vi "Exercise2.3-WBFM Modulation Demo (Music) .vi"() -> ()   [LabVIEW 2013]
uses:
  <vilib>/sound2/lvsound2.llb/Sound File Info (path).vi
  <vilib>/sound2/lvsound2.llb/Sound File Read Open.vi
  <vilib>/sound2/lvsound2.llb/Sound File Read (DBL).vi
  <vilib>/Waveform/WDTOps.llb/WDT Get Waveform Subset DBL.vi
  <vilib>/addons/Modulation/Analog/MT Passband PLL.vi
  <vilib>/express/express analysis/Spectral/Block/exnSpectralBlock spectral measurements power poly.vi
  <vilib>/express/express analysis/Spectral/Block/exnSpectralBlock spectral measurements power DDT.vi
  <vilib>/express/express analysis/Spectral/XNode/ExpressSpectralMeasurementsBlockNode.xnode
  <vilib>/addons/Modulation/niAMT.lvlib
  <vilib>/Analysis/NI_AALPro.lvlib
panel:
  out "Baseband":dynamicdata(graph)
  in  "Resample Rate":dbl=1000000.0 format="%#_13g"
  in  "Duration":dbl=44101.0 format="%#_13g"
  in  "path":path=path "D:/File/mozart.wav"
  out "Estimated freq.":dbl
  in  "WAV SR":dbl=44100.0 caption="dt"
  in  "LPF Cut-Off":dbl=60000.0 caption="Lower Cut-Off"
  in  "SNR (dB)":dbl(slide)=30.0 caption="Standard deviation" scale=-20.0..100.0
  out "Recovered Signal":dynamicdata(graph)
  out "FM Spectrum":dynamicdata(graph)
  out "FM Wave":dynamicdata(graph)
  in  "Carrier Amp.":dbl=1.0 caption="Amplitude"
  in  "stop":bool
  in  "Frequency Deviation":dbl(slide)=200.0 scale=0.0..100000.0
  in  "Carrier Freq.":dbl=100000.0 caption="Frequency"
  # "Frequency Modulation"
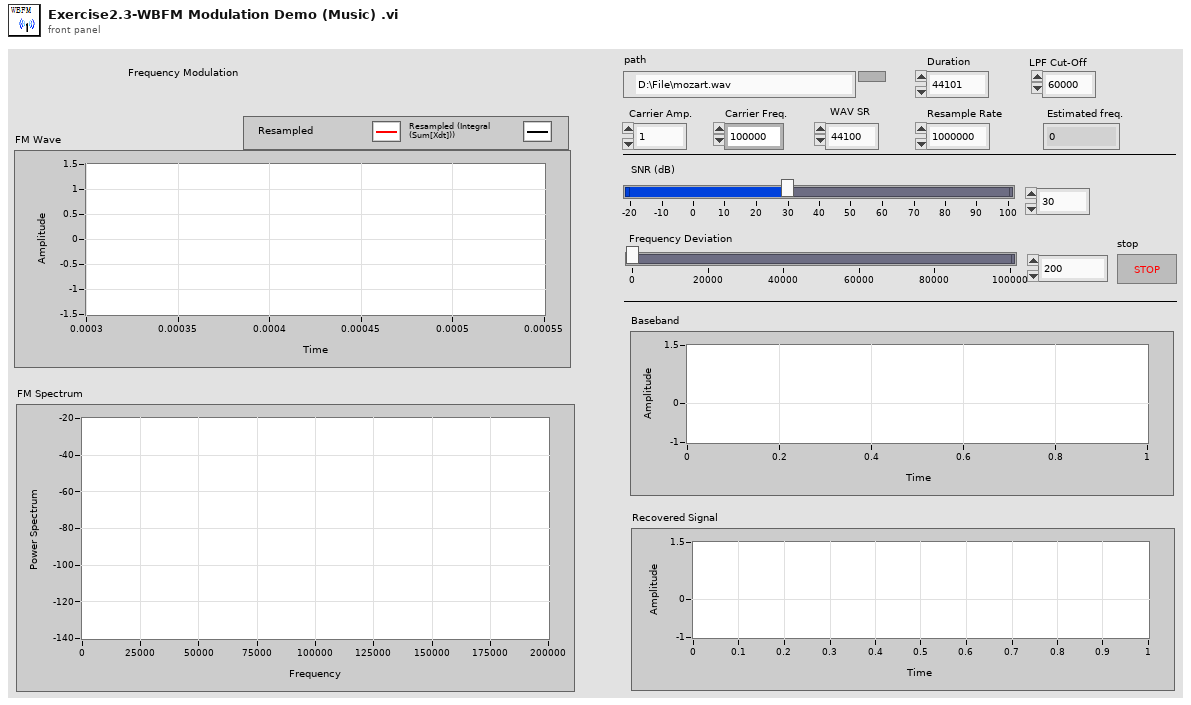
[diagram p1: front panel]
types:
  T1 = typedef "Sound File Refnum.ctl" = refnum<file>
  T2 = cluster{"averaging mode":u16, "weighting mode":u16, "number of averages":u32}
  T3 = cluster{"dB On (F)":bool, "unwrap phase (F)":bool, "convert to degree (F)":bool}
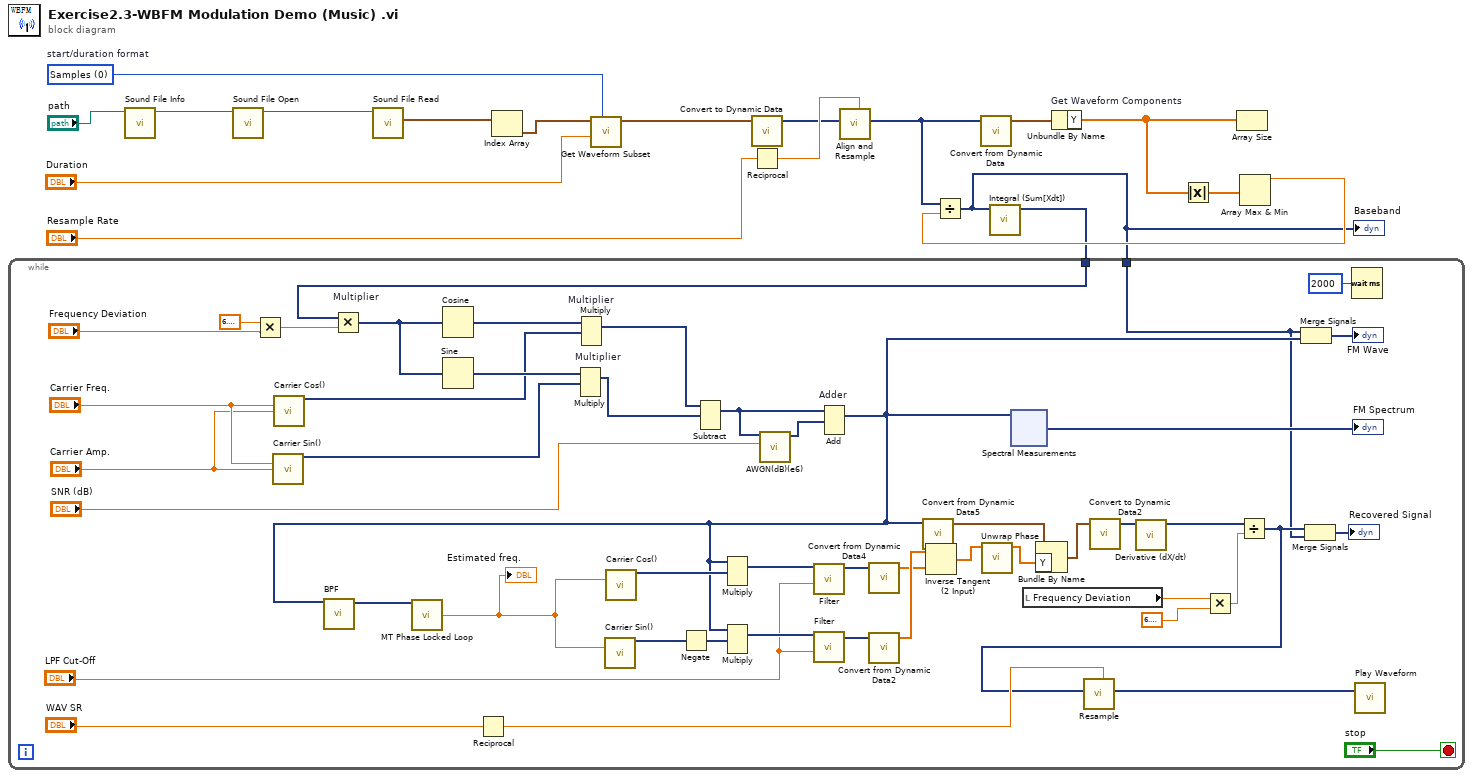
[diagram p0: block diagram]
diagram:
  w13 = u16 0 items=["Samples", "Relative Time"]  # start/duration format
  n1 = call-poly <vilib>:"Sound File Info.vi"("path"="path") -> ("path out"=w15:path)  [unwired: 7 in, 3 out]
  n2 = call-poly <vilib>:"Sound File Open.vi"("path"=w15) -> ("sound file refnum"=w18:T1)  [unwired: 9 in, 1 out]
  n3 = call-poly <vilib>:"Sound File Read.vi"("sound file refnum"=w18) -> ("data"=w17:waveform(dbl)[])  [unwired: 6 in, 4 out]
  n4 = Index Array "Index Array"(array=w17) -> (element=w6:waveform(dbl))  [unwired: 1 in]
  n5 = call-poly <vilib>:"Get Waveform Subset.vi"("start/duration format"=w13, "duration"="Duration", "waveform in"=w6) -> ("waveform out"=w10:waveform(dbl))  [unwired: 3 in, 3 out]
  n6 = call "Convert to Dynamic Data"("Waveform"=w10) -> ("Dynamic Data Type"=w5:dynamicdata)  [unwired: 3 in]
  n7 = Reciprocal(x="Resample Rate") -> (1/x=w11:dbl)
  n8 = call "Align and Resample"("dt"=w11, "Signals"=w5) -> ("Resampled Signals"=w3:dynamicdata)  [unwired: 7 in, 2 out]
  n9 = call "Convert from Dynamic Data"("Dynamic Data Type"=w3) -> ("Waveform"=w9:waveform(dbl))  [unwired: 3 in]
  n10 = Unbundle By Name "Get Waveform Components"(w9) -> ("Y"=w7:dbl[])
  n11 = Absolute Value(x=w7) -> (abs(x)=w8:dbl[])
  n12 = Array Size(array=w7) -> ()  [unwired: 1 out]
  n13 = Array Max & Min(array=w8) -> (max value=w4:dbl)  [unwired: 3 out]
  n14 = Divide(x=w3, y=w4) -> (x/y=w1:dynamicdata)
  "Baseband" <- w1
  n15 = call "Integral (Sum[Xdt])"("Signals"=w1) -> ("Result"=w2:dynamicdata)  [unwired: 5 in, 1 out]
  n16 = while {
    tunnel: w2 -> [w36]
    tunnel: w1 -> [w23]
    stop <- "stop" stop-if-true
    n17 = Multiply(x=6.283185307179586, y="Frequency Deviation") -> (x*y=w63:dbl)
    n18 = call "Carrier Sin()"("Frequency"="Carrier Freq.", "Amplitude"="Carrier Amp.") -> ("Sine"=w62:dynamicdata)  [unwired: 12 in, 1 out]
    n19 = call "Carrier Cos()"("Frequency"="Carrier Freq.", "Amplitude"="Carrier Amp.") -> ("Sine"=w45:dynamicdata)  [unwired: 12 in, 1 out]
    n20 = Multiply "Multiplier"(x=w36, y=w63) -> (x*y=w59:dynamicdata)
    n21 = Cosine(x=w59) -> (cos(x)=w46:dynamicdata)
    n22 = Sine(x=w59) -> (sin(x)=w51:dynamicdata)
    n23 = Reciprocal(x="WAV SR") -> (1/x=w43:dbl)
    n24 = Multiply "Multiplier"(1:w62, 2:w51) -> (0:w58:dynamicdata)  [unwired: 1 in, 1 out]
    n25 = Multiply "Multiplier"(1:w45, 2:w46) -> (0:w44:dynamicdata)  [unwired: 1 in, 1 out]
    n26 = Subtract(1:w58, 2:w44) -> (0:w57:dynamicdata)  [unwired: 1 in, 1 out]
    n27 = call "AWGN(dB)(e6).vi"("AWGN (dB)"="SNR (dB)", "Dynamic Data"=w57) -> ("DC with Gaussian Noise"=w61:dynamicdata)  [unwired: 9 in]
    n28 = Add "Adder"(1:w61, 2:w57) -> (0:w38:dynamicdata)  [unwired: 1 in, 1 out]
    n29 = call "BPF"("Signal"=w38) -> ("Filtered Signal"=w60:dynamicdata)  [unwired: 9 in, 1 out]
    n30 = call-poly <vilib>:"MT Phase Locked Loop.vi"("passband waveform"=w60) -> ("estimated carrier frequency (Hz)"=w27:dbl)  [unwired: 10 in, 4 out]
    "Estimated freq." <- w27
    n31 = call "Carrier Sin()"("Frequency"=w27) -> ("Sine"=w54:dynamicdata)  [unwired: 13 in, 1 out]
    n32 = call "Carrier Cos()"("Frequency"=w27) -> ("Sine"=w56:dynamicdata)  [unwired: 13 in, 1 out]
    n33 = Negate(x=w54) -> (-x=w53:dynamicdata)
    n34 = Multiply(1:w56, 2:w38) -> (0:w47:dynamicdata)  [unwired: 1 in, 1 out]
    n35 = Multiply(1:w53, 2:w38) -> (0:w55:dynamicdata)  [unwired: 1 in, 1 out]
    n36 = call "Filter"("Lower Cut-Off"="LPF Cut-Off", "Signal"=w47) -> ("Filtered Signal"=w37:dynamicdata)  [unwired: 8 in, 1 out]
    n37 = call "Filter"("Lower Cut-Off"="LPF Cut-Off", "Signal"=w55) -> ("Filtered Signal"=w52:dynamicdata)  [unwired: 8 in, 1 out]
    n38 = call "Convert from Dynamic Data4"("Dynamic Data Type"=w37) -> ("Array"=w49:dbl[])  [unwired: 3 in]
    n39 = call "Convert from Dynamic Data2"("Dynamic Data Type"=w52) -> ("Array"=w50:dbl[])  [unwired: 3 in]
    n40 = call "Convert from Dynamic Data5"("Dynamic Data Type"=w38) -> ("Waveform"=w41:waveform(dbl))  [unwired: 3 in]
    n41 = Inverse Tangent (2 Input)(1:w49, 2:w50) -> (0:w48:dbl[])
    n42 = call <vilib>:"Unwrap Phase.vi"("Phase"=w48) -> ("Unwrapped Phase"=w42:dbl[])  [unwired: 9 in, 1 out]
    n43 = xnode "Spectral Measurements"("Signals"=w38) -> ("Power Spectrum"=→"FM Spectrum":dynamicdata)  [unwired: 1 in, 1 out]
    n44 = local read "Frequency Deviation"() -> (w21:dbl)
    n45 = Bundle By Name(cluster=w41, "Y"=w42) -> (w40:waveform(dbl))
    n46 = call "Convert to Dynamic Data2"("Waveform"=w40) -> ("Dynamic Data Type"=w39:dynamicdata)  [unwired: 3 in]
    n47 = call "Derivative (dX/dt)"("Signals"=w39) -> ("Result"=w25:dynamicdata)  [unwired: 5 in, 1 out]
    n48 = Multiply(x=w21, y=6.283185307179586) -> (x*y=w19:dbl)
    n49 = Divide(x=w25, y=w19) -> (x/y=w24:dynamicdata)
    n50 = call "Resample"("dt"=w43, "Signals"=w24) -> ("Resampled Signals"=w22:dynamicdata)  [unwired: 7 in, 2 out]
    n51 = Merge Signals(w23, w38) -> (→"FM Wave":dynamicdata)
    n52 = Merge Signals(w24, w23) -> (→"Recovered Signal":dynamicdata)
    n53 = Wait (ms)(milliseconds to wait=u32 2000) -> ()  [unwired: 1 out]
    n54 = call "Play Waveform"("Data"=w22) -> ()  [unwired: 18 in, 1 out]
  }
